vi "Logger.vi"(7 "SaveLog?":bool, 8 "Input":dbl[](array[numeric]), 9 "Units Array":string[](array[string]), 10 "Errors Array":bool[](array[boolean]), 11 "selected path in":path) -> ()   [LabVIEW 2020]
uses:
  <vilib>/Utility/file.llb/Write To Spreadsheet File (string).vi
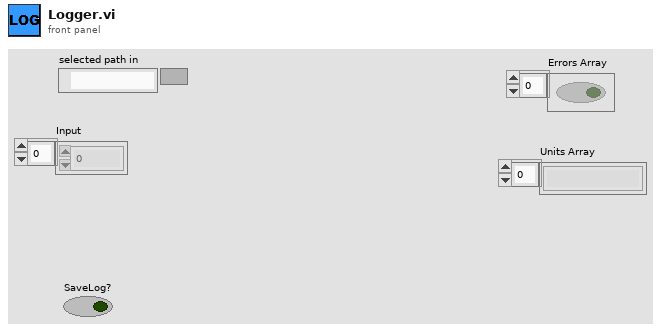
[diagram p1: front panel]
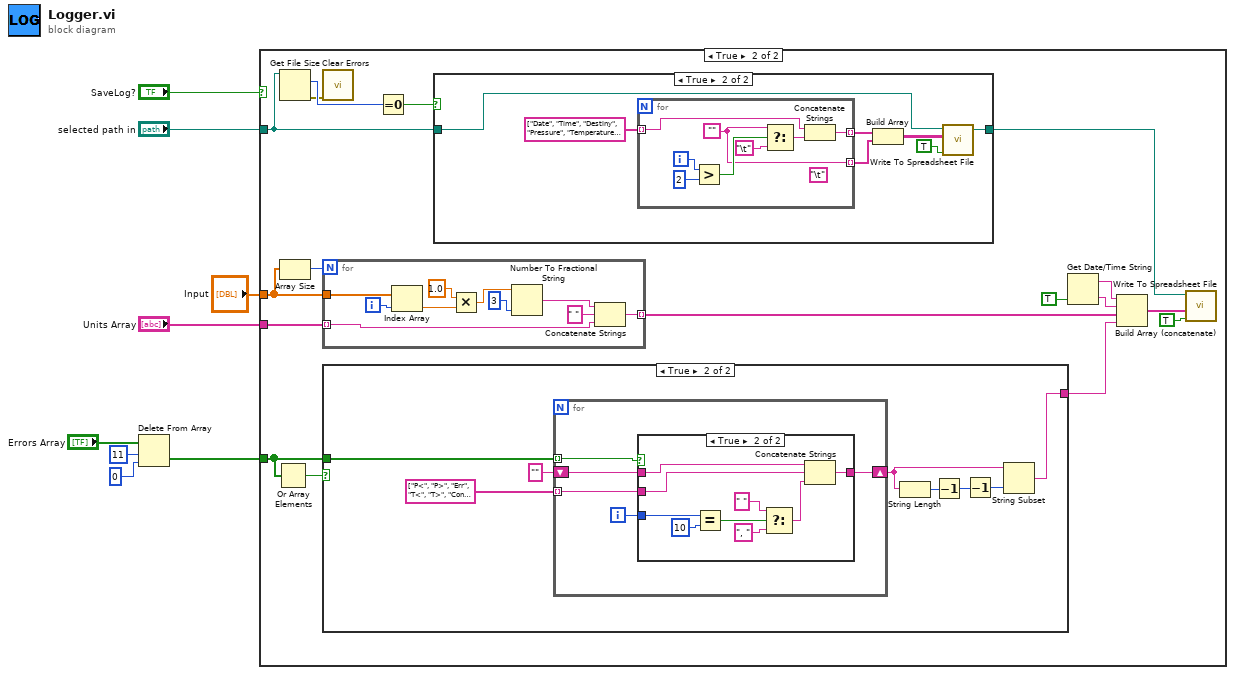
[diagram p0: block diagram]
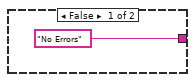
[diagram p4: hidden frame]
diagram:
  n1 = Delete From Array(array="Errors Array", length=11, index=0) -> (deleted portion=w1:bool[])  [unwired: 1 out]
  n2 = case shown="True" "SaveLog?" {
    tunnel: "selected path in" -> [_ w12]
    tunnel: "Input" -> [_ w25]
    tunnel: "Units Array" -> [_ w17]
    tunnel: w1 -> [_ w9]
    frame False {
    }
    frame True {
      n3 = Or Array Elements(Boolean array=w9) -> (logical OR=w16:bool)
      n4 = Get File Size(file=w12) -> (size (in bytes)=w13:i64, 0:w10:errorcluster)  [unwired: 1 in, 1 out]
      n5 = Array Size(array=w25) -> (size(s)=w24:i32)
      n6 = call <vilib>:"Clear Errors.vi"("error in (no error)"=w10) -> ()  [unwired: 5 in, 2 out]
      n7 = for {
        N: w24 -> [_]
        tunnel: w25 -> [w75]
        tunnel: [w66] -> w20 mode=indexing
        tunnel: w17 -> [w67] mode=indexing
        i -> [w74]
        n8 = Index Array(array=w75, index=w74) -> (element=w72:dbl)
        n9 = Multiply(x=1.0, y=w72) -> (x*y=w73:dbl)
        n10 = Number To Fractional String(number=w73, precision (6)=i16 3) -> (F-format string=w69:string)  [unwired: 2 in]
        n11 = Concatenate Strings(w69, " " ("string"), w67) -> (w66:string)
      }
      n12 = case shown="True" w16 {
        tunnel: w9 -> [_ w50]
        tunnel: ["No Errors" w46] -> w15
        frame False {
        }
        frame True {
          n13 = for {
            tunnel: w50 -> [w55] mode=indexing
            tunnel: string[] ["P<", "P>", "Err", "T<", "T>", "Conn ", "D<", "D>", "Err H", "Conn H", "MB"] -> [w54] mode=indexing
            shift-right: [w52] -> w47
            shift-left: "" -> [w53]
            i -> [w51]
            n14 = case shown="True" w55 {
              tunnel: w54 -> [_ w63]
              tunnel: w53 -> [w56 w65]
              tunnel: [w56 w64] -> w52
              tunnel: w51 -> [_ w62]
              frame False {
              }
              frame True {
                n15 = Equal?(x=w62, y=10) -> (x = y?=w60:bool)
                n16 = Select(t=" ", s=w60, f=", ") -> (s? t:f=w58:string)
                n17 = Concatenate Strings(w65, w63, w58) -> (w64:string)
              }
            }
          }
          n18 = String Length(string=w47) -> (length=w45:i32)
          n19 = Decrement(x=w45) -> (x-1=w44:i32)
          n20 = Decrement(x=w44) -> (x-1=w43:i32)
          n21 = String Subset(string=w47, length (rest)=w43) -> (substring=w46:string)  [unwired: 1 in]
        }
      }
      n22 = Equal To 0?(x=w13) -> (x = 0?=w14:bool)
      n23 = case shown="True" w14 {
        tunnel: w12 -> [w26 w32]
        tunnel: [w26 w31] -> w11
        frame False {
        }
        frame True {
          n24 = for {
            tunnel: string[] ["Date", "Time", "Destiny", "Pressure", "Temperature", "Reduced P.", "Errors"] -> [w41] mode=indexing
            tunnel: [w40] -> w29 mode=indexing
            tunnel: [w34] -> w28 mode=indexing
            i -> [w39]
            w34 = ""
            (unwired) "\t"
            n25 = Greater?(x=w39, y=2) -> (0:w37:bool)
            n26 = Select(t=w34, s=w37, f="\t") -> (s? t:f=w35:string)
            n27 = Concatenate Strings(w41, w35) -> (w40:string)
          }
          n28 = Build Array(w29, w28) -> (w27:string[][])
          n29 = call-poly <vilib>:"Write To Spreadsheet File.vi"("append to file? (new file:F)"=TRUE, "2D data"=w27, "file path (dialog if empty)"=w32) -> ("new file path (Not A Path if cancelled)"=w31:path)  [unwired: 5 in]
        }
      }
      n30 = Get Date/Time String(want seconds? (F)=TRUE) -> (date string=w21:string, time string=w22:string)  [unwired: 2 in]
      n31 = Build Array (concatenate)(w21, w22, w20, w15) -> (w18:string[])
      n32 = call-poly <vilib>:"Write To Spreadsheet File.vi"("append to file? (new file:F)"=TRUE, "1D data"=w18, "file path (dialog if empty)"=w11) -> ()  [unwired: 5 in, 1 out]
    }
  }
